vi "SRV_Build Sensor-Value Cluster.vi"(0 "Cfg-Cmds":T3[](array[typedef]) {"Calculated Sensors Array"."Parsed Formula"."Y Values" format="%.2f"; "Calculated Sensors Array"."Sensor Config"."Register" format="%.0x"; "Calculated Sensors Array"."Sensor Config"."I2C Address" format="%.0x"; "Calculated Sensors Array"."Sensor Config"."Sample Period (ms)" min=10 max=60000 step=1; "Calculated Sensors Array"."Sensor Config"."Digital Mask" format="%.0x"; "Calculated Sensors Array"."Sensor Config"."Channel" format="%.0x"; "Parsed Formula"."Y Values" format="%.2f"; "Sensor Config"."Register" format="%.0x"; "Sensor Config"."I2C Address" format="%.0x"; "Sensor Config"."Sample Period (ms)" min=10 max=60000 step=1; "Sensor Config"."Digital Mask" format="%.0x"; "Sensor Config"."Channel" format="%.0x"}, 5 "Sensor View Indicator Names":T1[](array[typedef]), 7 "Sensor View Indicator Name":T1, 9 "Value (for Pico C)":dbl=nan, 11 "error in (no error)":errorcluster, 12 "Value (U16)":u16, 13 "Value (U8)":u8) -> (8 "Array of Sensor-Value Cluster":T2[](array[typedef]), 15 "error out":errorcluster)   [LabVIEW 2014]
uses:
  SRV_Sensor Config-Command Cluster.ctl
  SRV_Sensor Config Cluster.ctl
  SRV_Sensor Analog-Digital.ctl
  SRV_Sensor Sampling Mode.ctl
  SRV_Sensor View Config Cluster.ctl
  SRV_Sensors Names.ctl
  SRV_Sensor PicoC Shared Var Type.ctl
  SRV_Sensor Number of Bytes.ctl
  SRV_Sensor Integer Word Type.ctl
  SRV_Calculated Sensor Cfg.ctl
  SRV_Sensor-Value Cluster.ctl
panel:
  # "operator"
  # "register1"
  # "register2"
  # "operator"
  # "register1"
  # "register2"
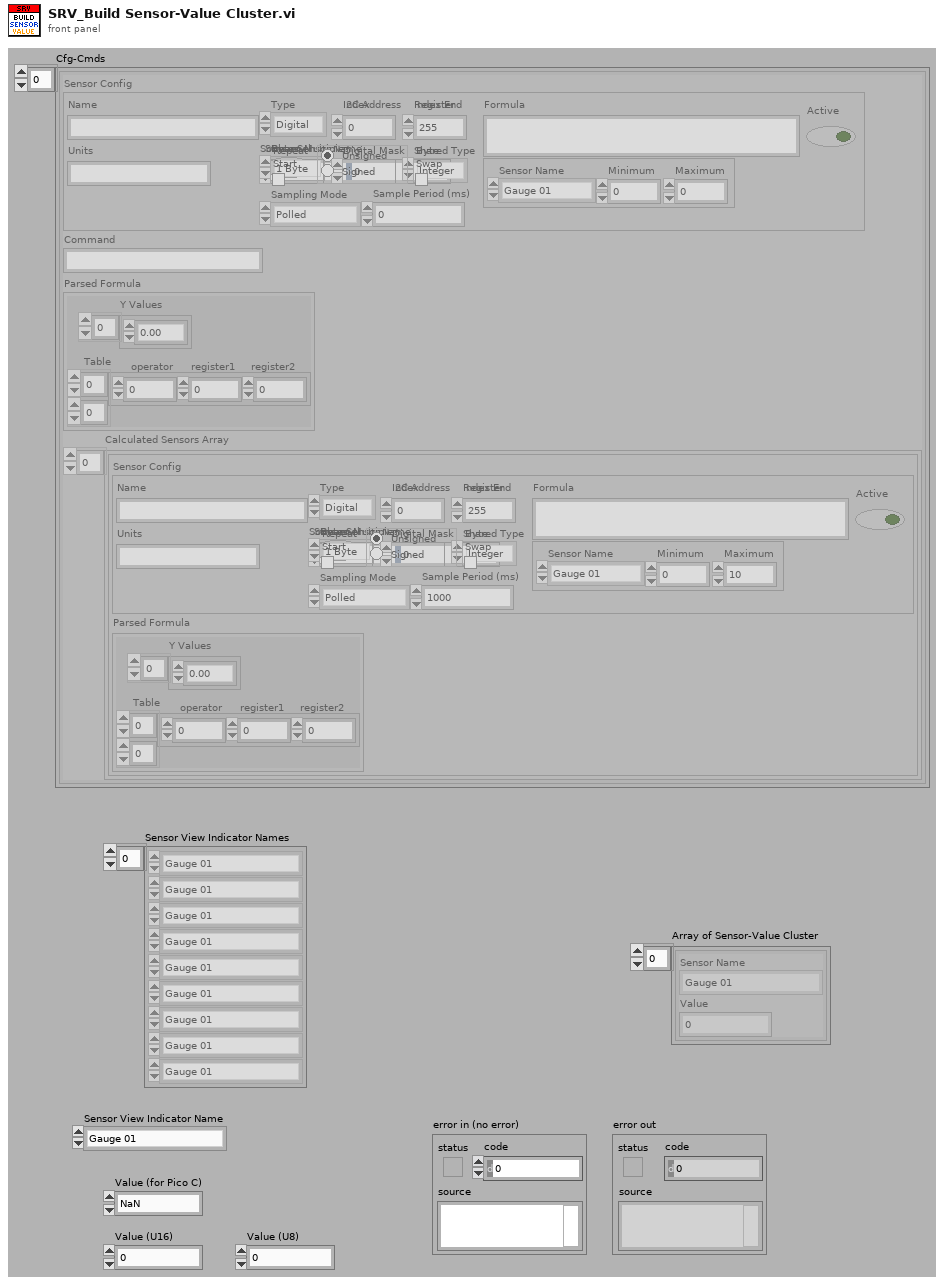
[diagram p1: front panel]
types:
  T1 = typedef "SRV_Sensors Names.ctl" = enum16{"Gauge 01", "Gauge 02", "Gauge 03", "Gauge 04", "Meter 01", "Meter 02", "Meter 03", "Meter 04", "Numeric 01", "Numeric 02", "Numeric 03", "Numeric 04", "Numeric 05", "Numeric 06", "Numeric 07", "Numeric 08", "Boolean 01", "Boolean 02", "Boolean 03", "Boolean 04", "Boolean 05", "Boolean 06", "Boolean 07", "Boolean 08", "Boolean 09", "Boolean 10", "Boolean 11", "Boolean 12", "Boolean 13", "Boolean 14", "Boolean 15", "Boolean 16", "Boolean 17", "Boolean 18", "Boolean 19", "Boolean 20", "Boolean 21", "Boolean 22", "Boolean 23", "Boolean 24", "Boolean 25", "Boolean 26", "Boolean 27", "Boolean 28", "Boolean 29", "Boolean 30", "Boolean 31", "Boolean 32"}
  T2 = typedef "SRV_Sensor-Value Cluster.ctl" = cluster{"Sensor Name":T1, "Value":dbl}
  T3 = typedef "SRV_Sensor Config-Command Cluster.ctl" = cluster{"Sensor Config":T4, "Command":string, "Parsed Formula":cluster{"Table":i32[][], "Y Values":dbl[]}, "Calculated Sensors Array":T11[]}
  T4 = typedef "SRV_Sensor Config Cluster.ctl" = cluster{"Name":string, "A/D":T5, "I2C Address":u8, "Register":u8, "Channel":u8, "Digital Mask":u16, "Units":string, "Sampling Mode":T6, "Sample Period (ms)":u32, "Formula":string, "Sensor View Config":T7, "Active":bool, "PicoC Shared Var Type":T8, "Index":u8, "Stream Multiple?":bool, "Index End":u8, "Bytes":T9, "Source Sensor Name":string, "Repeat Start":bool, "Integer Word Type":T10, "Byte Swap":bool}
  T5 = typedef "SRV_Sensor Analog-Digital.ctl" = enum16{"Digital", "Analog", "PicoC Shared", "Calculated"}
  T6 = typedef "SRV_Sensor Sampling Mode.ctl" = enum16{"Polled", "Streaming"}
  T7 = typedef "SRV_Sensor View Config Cluster.ctl" = cluster{"Sensor Name":T1, "Minimum":dbl, "Maximum":dbl}
  T8 = typedef "SRV_Sensor PicoC Shared Var Type.ctl" = enum16{"String", "Integer", "Float"}
  T9 = typedef "SRV_Sensor Number of Bytes.ctl" = enum16{"1 Byte", "2 Bytes"}
  T10 = typedef "SRV_Sensor Integer Word Type.ctl" = enum32{"Unsigned", "Signed"}
  T11 = typedef "SRV_Calculated Sensor Cfg.ctl" = cluster{"Sensor Config":T4, "Parsed Formula":cluster{"Table":i32[][], "Y Values":dbl[]}}
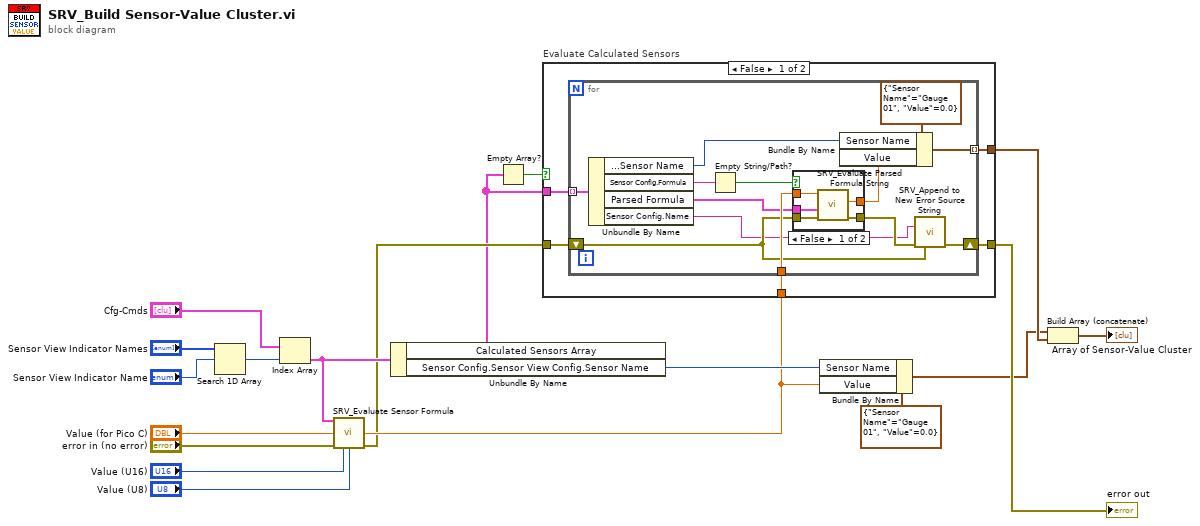
[diagram p0: block diagram]
diagram:
  n1 = Search 1D Array(1D array="Sensor View Indicator Names", element="Sensor View Indicator Name") -> (index of element=w1:i32)  [unwired: 1 in]
  n2 = Index Array(array="Cfg-Cmds", index=w1) -> (element=w8:T3)
  n3 = call "SRV_Evaluate Sensor Formula.vi"("Sensor Cfg-Command Cluster"=w8, "Value"="Value (for Pico C)", "error in (no error)"="error in (no error)", "Value (U16)"="Value (U16)", "Value (U8)"="Value (U8)") -> ("Value out"=w7:dbl, "error out"=w6:errorcluster)  [unwired: 9 in]
  n4 = Unbundle By Name(w8) -> ("Calculated Sensors Array"=w3:T11[], "Sensor Config.Sensor View Config.Sensor Name"=w10:T1)
  n5 = Empty Array?(array=w3) -> (empty?=w2:bool)
  n6 = case "Evaluate Calculated Sensors" shown="False" w2 {
    tunnel: w7 -> [w24 _]
    tunnel: w3 -> [w23 _]
    tunnel: w6 -> [w22 w45]
    tunnel: [w21 w45] -> w17
    tunnel: [w20 _] -> w5
    frame False {
      n7 = for {
        tunnel: w24 -> [w34]
        tunnel: w23 -> [w37] mode=indexing
        shift-right: [w30] -> w21
        shift-left: w22 -> [w32]
        tunnel: [w25] -> w20 mode=indexing
        n8 = Unbundle By Name(w37) -> ("Sensor Config.Sensor View Config.Sensor Name"=w27:T1, "Sensor Config.Formula"=w36:string, "Parsed Formula"=w33:cluster{"Table":i32[][], "Y Values":dbl[]}, "Sensor Config.Name"=w29:string)
        n9 = Empty String/Path?(string/path=w36) -> (empty?=w35:bool)
        n10 = case shown="False" w35 {
          tunnel: w33 -> [w42 _]
          tunnel: w32 -> [w41 w43]
          tunnel: [w40 w43] -> w31
          tunnel: [w39 w44] -> w26
          tunnel: w34 -> [w38 w44]
          frame False {
            n11 = call "SRV_Evaluate Parsed Formula String.vi"("error in (no error)"=w41, "Parsed Formula"=w42, "Variable v"=w38) -> ("error out"=w40:errorcluster, "Value out"=w39:dbl)  [unwired: 7 in]
          }
          frame True {
          }
        }
        n12 = Bundle By Name(cluster=T2 {"Sensor Name"=enum."Gauge 01", "Value"=0.0} ("Sensor-Value Cluster"), "Sensor Name"=w27, "Value"=w26) -> (w25:T2)
        n13 = call "SRV_Append to New Error Source String.vi"("Message String to append"=w29, "Error In (no error)"=w31, "Previous Error In (no error)"=w32) -> ("error out"=w30:errorcluster)  [unwired: 12 in]
      }
    }
    frame True {
    }
  }
  "error out" <- w17
  n14 = Bundle By Name(cluster=T2 {"Sensor Name"=enum."Gauge 01", "Value"=0.0} ("Sensor-Value Cluster"), "Sensor Name"=w10, "Value"=w7) -> (w4:T2)
  n15 = Build Array (concatenate)(w4, w5) -> (→"Array of Sensor-Value Cluster":T2[])
